vi "LaserKoherasGetFGV.vi"(10 "Set_Get":enum16{"Set", "Get"}(ring), 11 "LaserVarSet":string[](array[string])) -> (3 "LaserVarGet":string[](array[string]))   [LabVIEW 2010]
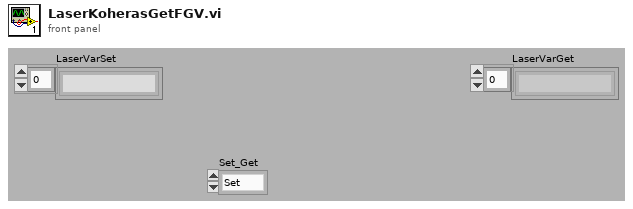
[diagram p1: front panel]
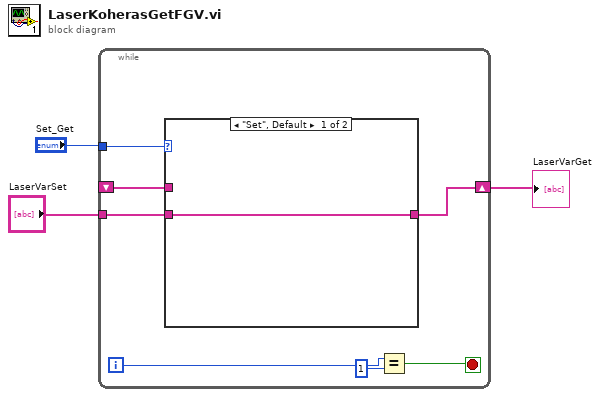
[diagram p0: block diagram]
diagram:
  n1 = while {
    tunnel: "Set_Get" -> [w10]
    tunnel: "LaserVarSet" -> [w9]
    shift-right: [w8] -> w2
    shift-left: _ -> [w7]
    i -> [w5]
    stop <- w6 stop-if-true
    n2 = case shown="\"Set\", Default" w10 {
      tunnel: w9 -> [w11 _]
      tunnel: [w11 w12] -> w8
      tunnel: w7 -> [_ w12]
      frame "Set", Default {
      }
      frame "Get" {
      }
    }
    n3 = Equal?(x=w5, y=1) -> (x = y?=w6:bool)
  }
  "LaserVarGet" <- w2
